vi "Update DynData in MeasDataQ.vi"(4 "UpdateTS (T)":bool=TRUE, 8 "error in (no error)":errorcluster, 9 "TimeStamp":timestamp, 10 "CurrentDyn":dbl, 11 "VoltageDyn":dbl) -> (0 "error out":errorcluster, 3 "orData out":T1)   [LabVIEW 2017]
doc: "Developed by Kevin Thompson\nThompson Engineering, LLC\nkevin@thompsonengineering.net"
uses:
  TD MeasData QRef.ctl
  TD MeasData--cluster.ctl
  GBL DataQ Ref.vi
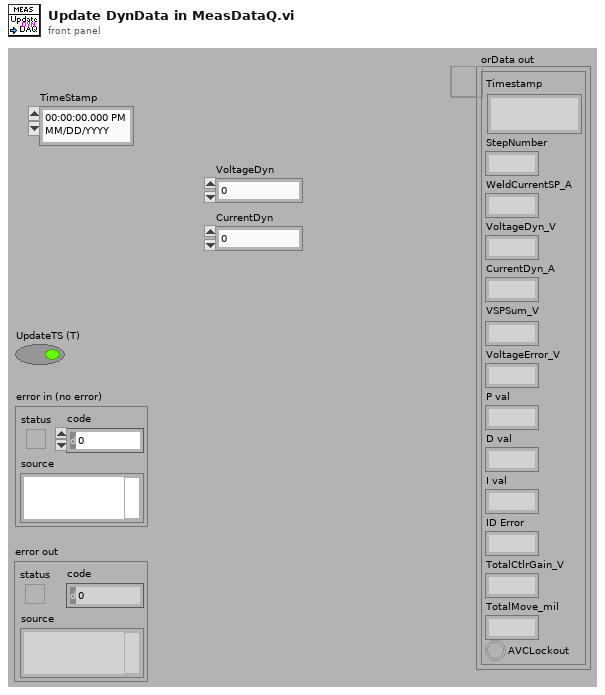
[diagram p1: front panel]
types:
  T1 = typedef "TD MeasData QRef.ctl" = refnum<queue>
  T2 = typedef "TD MeasData--cluster.ctl" = cluster{"Timestamp":timestamp, "StepNumber":i32, "WeldCurrentSP_A":dbl, "VoltageDyn_V":dbl, "CurrentDyn_A":dbl, "VSPSum_V":dbl, "VoltageError_V":dbl, "P val":dbl, "D val":dbl, "I val":dbl, "ID Error":dbl, "TotalCtlrGain_V":dbl, "TotalMove_mil":dbl, "AVCLockout":bool}
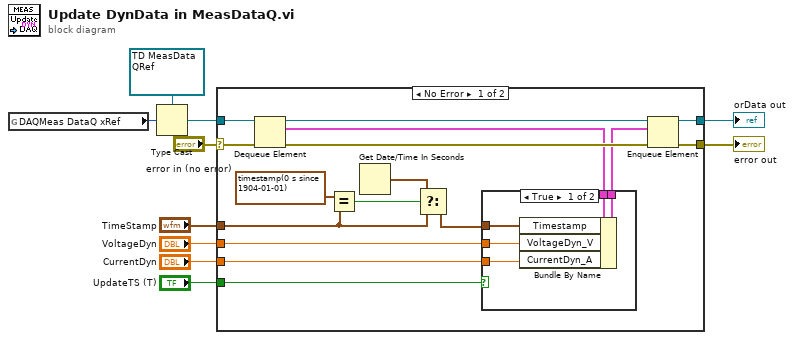
[diagram p0: block diagram]
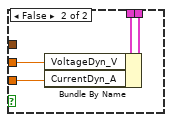
[diagram p2: hidden frame]
diagram:
  n1 = global read "GBL DataQ Ref.vi" "DAQMeas DataQ xRef"() -> (w4:u32)
  n2 = Type Cast(type=T1 refnum ("orData in"), x=w4) -> (*(type *) &x=w6:T1)
  n3 = case shown="No Error" "error in (no error)" {
    selector: "error in (no error)" -> [w21 w36]
    tunnel: w6 -> [w26 w37]
    tunnel: [w23 w36] -> w10
    tunnel: [w22 w37] -> w9
    tunnel: "TimeStamp" -> [w14 _]
    tunnel: "VoltageDyn" -> [w18 _]
    tunnel: "CurrentDyn" -> [w17 _]
    tunnel: "UpdateTS (T)" -> [w11 _]
    frame No Error {
      n4 = Dequeue Element(queue=w26, error in (no error)=w21) -> (queue out=w24:T1, element=w20:T2, error out=w25:errorcluster)  [unwired: 1 in, 1 out]
      n5 = Equal?(x=timestamp(0 s since 1904-01-01) ("TimeStamp"), y=w14) -> (x = y?=w15:bool)
      n6 = Get Date/Time In Seconds() -> (seconds since 1Jan1904=w12:timestamp)
      n7 = Select(t=w12, s=w15, f=w14) -> (s? t:f=w13:timestamp)
      n8 = case shown="True" w11 {
        tunnel: w20 -> [w31 w35]
        tunnel: [w30 w34] -> w19
        tunnel: w18 -> [w29 w33]
        tunnel: w17 -> [w28 w32]
        tunnel: w13 -> [w27 _]
        frame True {
          n9 = Bundle By Name(cluster=w31, "Timestamp"=w27, "VoltageDyn_V"=w29, "CurrentDyn_A"=w28) -> (w30:T2)
        }
        frame False {
          n10 = Bundle By Name(cluster=w35, "VoltageDyn_V"=w33, "CurrentDyn_A"=w32) -> (w34:T2)
        }
      }
      n11 = Enqueue Element(queue=w24, element=w19, error in (no error)=w25) -> (queue out=w22:T1, error out=w23:errorcluster)  [unwired: 1 in, 1 out]
    }
    frame Error {
    }
  }
  "orData out" <- w9
  "error out" <- w10
